vi "hex convert to_float.vi"() -> ()   [LabVIEW 2020]
panel:
  in  "Array 2":u8[](array[numeric]) format="%02x"
  out "float":dbl
  out "Array":u8[](array[numeric]) format="%x"
  in  "data[]":string[](array[string])=["00", "00", "00", "00"]
  out "float":sgl format="%#_13g"
  # "0x3d4ccccd"
  # "=> 0.05000000074506"
  # "0x461c4000"
  # "=>10000"
  # "0x42AA aa0000"
  # "=> 85"
  # "0xC1A00000"
  # "=>-20"
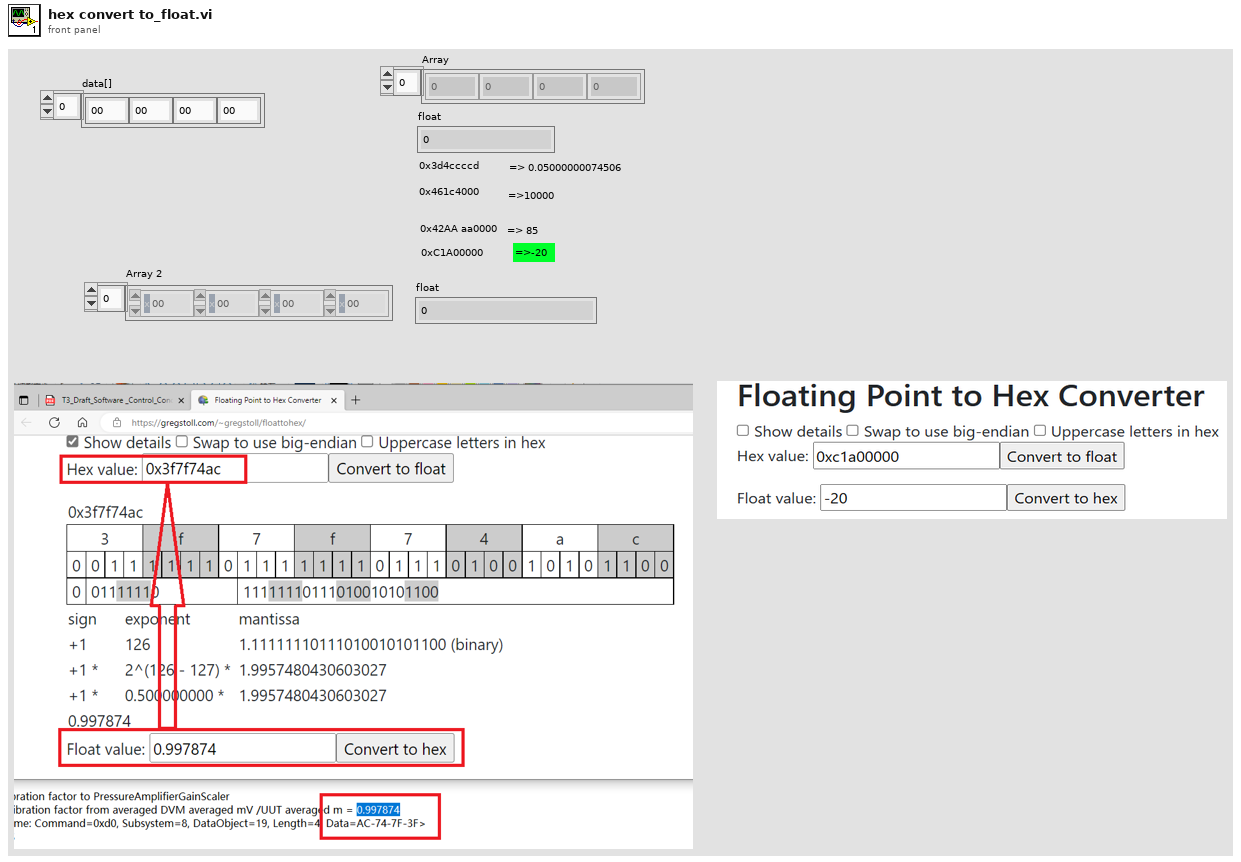
[diagram p1: front panel]
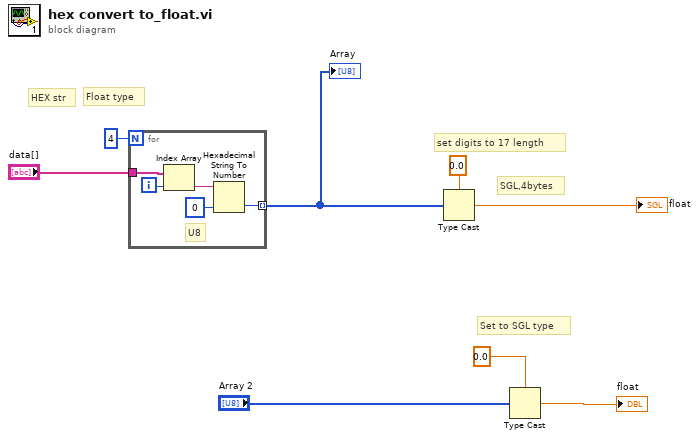
[diagram p0: block diagram]
diagram:
  # "Set to SGL type"
  # "SGL,4bytes"
  # "Float type"
  # "set digits to 17 length"
  # "HEX str"
  n1 = for {
    N: 4 -> [_]
    tunnel: [w11] -> w5 mode=indexing
    tunnel: "data[]" -> [w10]
    i -> [w13]
    # "U8"
    n2 = Index Array(array=w10, index=w13) -> (element=w9:string)
    n3 = Hexadecimal String To Number(string=w9, default (0uL)=u8 0 ("default (0 I32)")) -> (number=w11:u8)  [unwired: 1 in, 1 out]
  }
  "Array" <- w5
  n4 = Type Cast(type=sgl 0.0, x=w5) -> (*(type *) &x=→"float":sgl)
  n5 = Type Cast(type=sgl 0.0, x="Array 2") -> (*(type *) &x=→"float":sgl)
